vi "Arrays.vi"() -> ()   [LabVIEW 2019]
panel:
  out "element":dbl
  out "size(s)":i32
  in  "Array 3":bool[](array[boolean])
  out "Array 2":dbl[](array[numeric])
  in  "Array":dbl[](array[numeric])
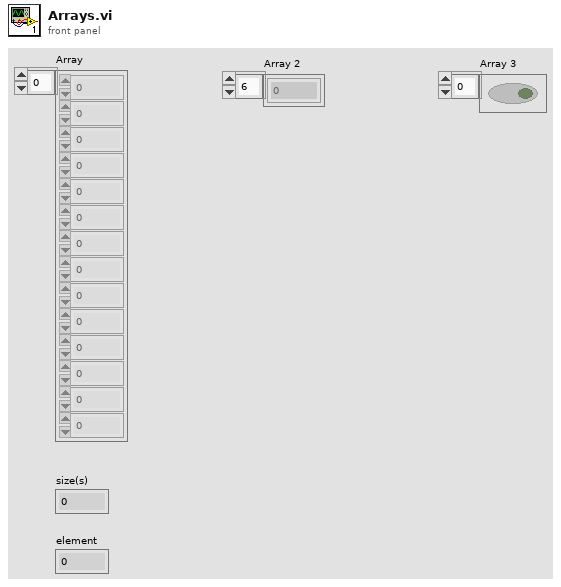
[diagram p1: front panel]
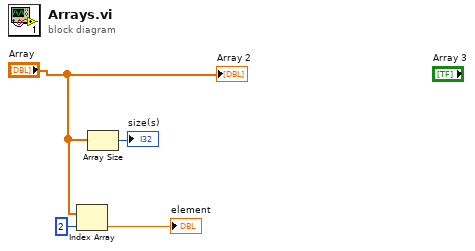
[diagram p0: block diagram]
diagram:
  n1 = Index Array(array="Array", index=2) -> (element=→"element":dbl)
  n2 = Array Size(array="Array") -> (size(s)=→"size(s)":i32)
  "Array 2" <- "Array"
